vi "串口通讯基本流程.vi"(3 "错误输入（无错误）":errorcluster, 4 "通讯参数":T1={"写入缓冲区"="+TXYBJT TECH", "等待时间（毫秒）"=500, "搜索字符串/字符(-)"="Software,VERdowa_v"}, 5 "串口设置":T2={"COM号"="COM1", "波特率"=9600, "数据比特"=8, "奇偶"=enum."None", "停止位"=10, "流控制"=0} {"流控制" items=["无"=0, "XON/XOFF"=1, "RTS/CTS"=2, "DTR/DSR"=4]; "停止位" items=["1.0"=10, "1.5"=15, "2.0"=20]; "波特率" items=["75"=75, "110"=110, "134"=134, "150"=150, "300"=300, "600"=600, "1200"=1200, "1800"=1800, "2400"=2400, "4800"=4800, "7200"=7200, "9600"=9600, "14400"=14400, "19200"=19200, "28800"=28800, "38400"=38400, "56000"=56000, "57600"=57600, "115200"=115200, "128000"=128000, "230400"=230400]}) -> (0 "错误输出":errorcluster, 1 "GetRightData？":bool, 2 "获取数据":string)   [LabVIEW 2015]
uses:
  Serial - Settings.ctl
  <vilib>/Instr/_visa.llb/VISA Configure Serial Port (Instr).vi
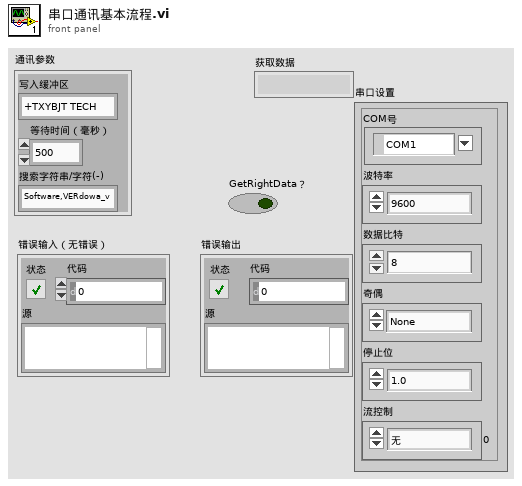
[diagram p1: front panel]
types:
  T1 = cluster{"写入缓冲区":string, "等待时间（毫秒）":u32, "搜索字符串/字符(-)":string}
  T2 = typedef "Serial - Settings.ctl" = cluster{"COM号":refnum<visa-resource-name>, "波特率":u32, "数据比特":u16, "奇偶":enum16{"None", "Odd", "Even", "Mark", "Space"}, "停止位":u16, "流控制":u16}
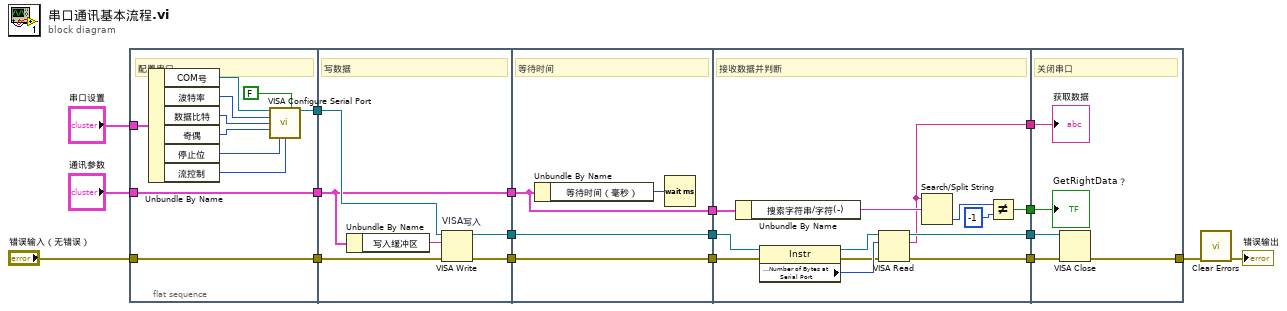
[diagram p0: block diagram]
diagram:
  n1 = flat-sequence {
    tunnel: "错误输入（无错误）" -> [w29]
    tunnel: [w20] -> w18
    tunnel: [w29] -> w17
    tunnel: "串口设置" -> [w28]
    tunnel: [w19] -> w5
    tunnel: "通讯参数" -> [w19]
    tunnel: [w33] -> w16
    tunnel: [w32] -> w15
    tunnel: w18 -> [w35]
    tunnel: w17 -> [w34]
    tunnel: w5 -> [w30]
    tunnel: [w30] -> w3
    tunnel: w16 -> [w39]
    tunnel: [w39] -> w14
    tunnel: [w38] -> w13
    tunnel: w15 -> [w38]
    tunnel: w3 -> [w36]
    tunnel: [w36] -> w2
    tunnel: w14 -> [w52]
    tunnel: w13 -> [w51]
    tunnel: [w47] -> w10
    tunnel: [w46] -> w9
    tunnel: [w43] -> w8
    tunnel: w2 -> [w41]
    tunnel: [w40] -> w1
    tunnel: [w54] -> w7
    tunnel: w10 -> [w56]
    tunnel: w9 -> [w55]
    tunnel: w8 -> [w57]
    tunnel: w1 -> [w53]
    frame #0 {
      # "配置串口"
      n2 = Unbundle By Name(w28) -> ("COM号"=w27:refnum<visa-resource-name>, "波特率"=w26:u32, "数据比特"=w25:u16, "奇偶"=w24:enum16{"None", "Odd", "Even", "Mark", "Space"}, "停止位"=w23:u16, "流控制"=w22:u16)
      n3 = call-poly "VISA Configure Serial Port"("VISA resource name"=w27, "Enable Termination\nChar (T)"=FALSE ("Enable Termination\nChar (T)"), "baud rate (9600)"=w26, "data bits (8)"=w25, "parity (0:none)"=w24, "stop bits (10: 1 bit)"=w23, "flow control (0:none)"=w22) -> ("VISA resource name out"=w20:refnum<visa-resource-name>)  [unwired: 7 in, 1 out]
    }
    frame #1 {
      # "写数据"
      n4 = Unbundle By Name(w30) -> ("写入缓冲区"=w31:string)
      n5 = VISA Write "VISA写入"(VISA resource name=w35, write buffer=w31, error in (no error)=w34) -> (VISA resource name out=w33:refnum<visa-resource-name>, error out=w32:errorcluster)  [unwired: 1 out]
    }
    frame #2 {
      # "等待时间"
      n6 = Unbundle By Name(w36) -> ("等待时间（毫秒）"=w37:u32)
      n7 = Wait (ms)(milliseconds to wait=w37) -> ()  [unwired: 1 out]
    }
    frame #3 {
      # "接收数据并判断"
      n8 = Unbundle By Name(w41) -> ("搜索字符串/字符(-)"=w42:string)
      n9 = property class="Instr"(reference=w52, error in=w51) -> (reference out=w49:refnum<visa-resource-name>, error out=w48:errorcluster, "Serial Settings:Number of Bytes at Serial Port"=w50:u32)
      n10 = VISA Read(VISA resource name=w49, byte count=w50, error in (no error)=w48) -> (VISA resource name out=w47:refnum<visa-resource-name>, read buffer=w40:string, error out=w46:errorcluster)  [unwired: 1 out]
      n11 = Search/Split String(string=w40, search string/char (-)=w42) -> (offset of match=w45:i32)  [unwired: 1 in, 2 out]
      n12 = Not Equal?(x=w45, y=-1) -> (x != y?=w43:bool)
    }
    frame #4 {
      # "关闭串口"
      n13 = VISA Close(VISA resource name=w56, error in (no error)=w55) -> (error out=w54:errorcluster)
      "GetRightData？" <- w57
      "获取数据" <- w53
    }
  }
  n14 = call <vilib>:"Clear Errors.vi"("error in (no error)"=w7) -> ("error out"=→"错误输出":errorcluster)  [unwired: 5 in, 1 out]
